vi "Section Page.vi"(8 "error in (no error)":errorcluster, 11 "Node Ptr":T1 format="%.0x") -> (0 "error out":errorcluster)   [LabVIEW 2019, in "Protection and Counter Addon System Explorer.lvlib"]
uses:
  Protection and Counter Addon System Explorer.lvlib
  <vilib>/NI VeriStand/Custom Device API/Custom Device Item Ref.ctl
  <vilib>/NI VeriStand/Custom Device API/Custom Device API.lvlib
panel:
  in  "SHDocVw.IWebBrowser2":refnum<k7>(container)
types:
  T1 = typedef "Custom Device API.lvlib/Custom Device Item Ref.ctl" = u64
  T2 = typedef "Custom Device API.lvlib/Custom Device Item Info.ctl" = cluster{"Name":string, "Is Channel":bool, "GUID":string, "Is Waveform":bool}
  T3 = typedef "Custom Device API.lvlib/Custom Device Commands.ctl" = enum16{"Default", "Item renamed", "Shutdown", "Dynamic button pressed"}
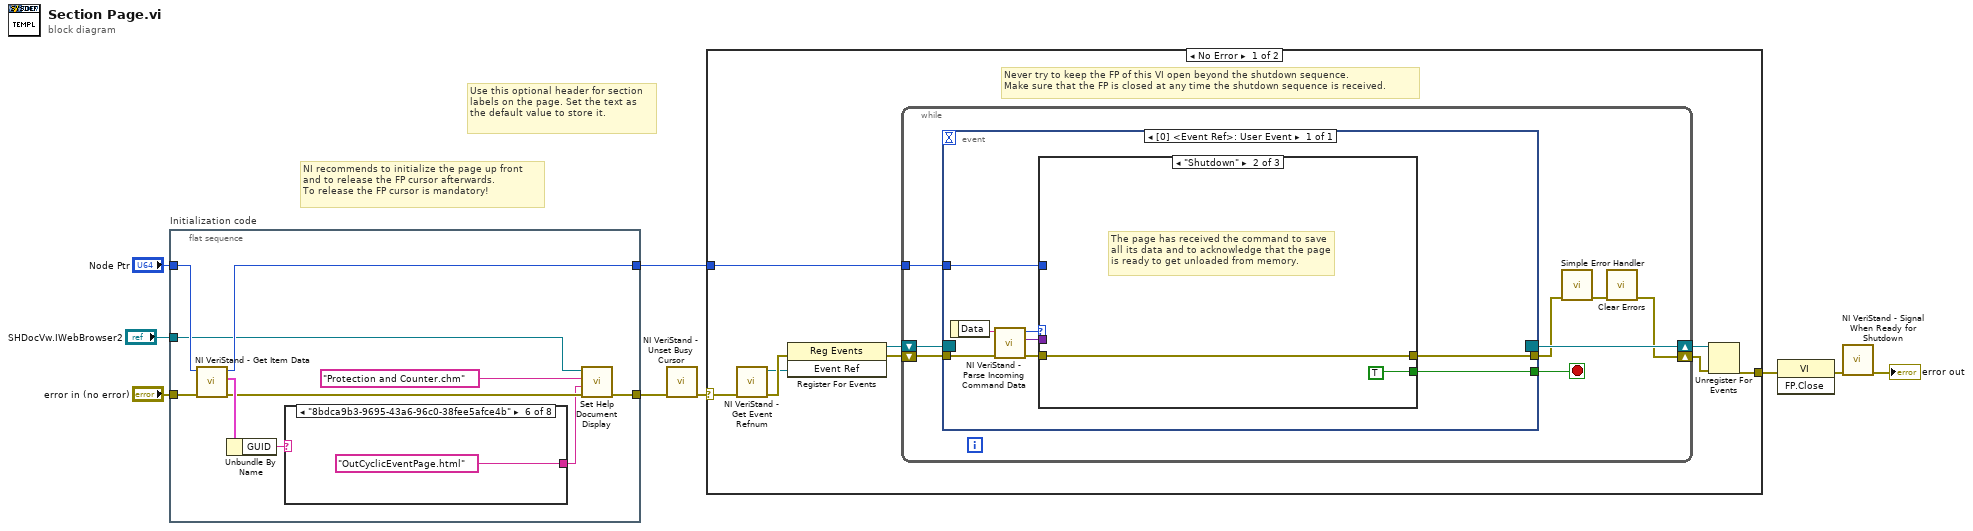
[diagram p0: block diagram]
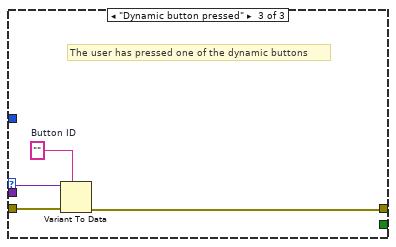
[diagram p3: hidden frame]
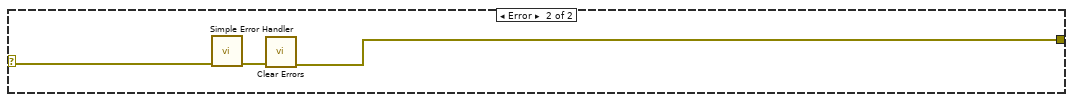
[diagram p4: hidden frame]
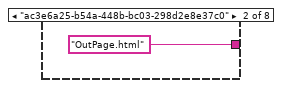
[diagram p6: hidden frame]
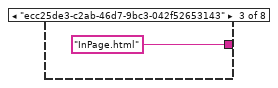
[diagram p7: hidden frame]
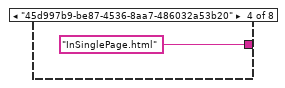
[diagram p8: hidden frame]
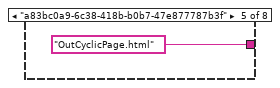
[diagram p9: hidden frame]
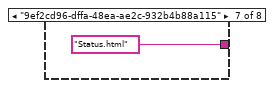
[diagram p10: hidden frame]
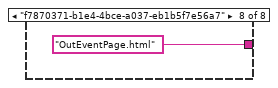
[diagram p11: hidden frame]
diagram:
  # "Use this optional header for section labels on the page. Set the text as the default value to store it."
  # "NI recommends to initialize the page up front\nand to release the FP cursor afterwards.\nTo release the FP cursor is mandatory!"
  n1 = flat-sequence "Initialization code" {
    tunnel: "error in (no error)" -> [w17]
    tunnel: "Node Ptr" -> [w19]
    tunnel: [w13] -> w5
    tunnel: [w18] -> w2
    tunnel: "SHDocVw.IWebBrowser2" -> [w10]
    frame #0 {
      n2 = call <vilib>:"NI VeriStand - Get Item Data.vi"("error in (no error)"=w17, "Item Ref in"=w19) -> ("error out"=w14:errorcluster, "Item Info"=w16:T2, "Item Ref out"=w18:T1)  [unwired: 6 in, 1 out]
      n3 = Unbundle By Name(w16) -> ("GUID"=w15:string)
      n4 = case shown="\"8bdca9b3-9695-43a6-96c0-38fee5afce4b\"" w15 {
        tunnel: [_ "OutPage.html" ("HTML File") "InPage.html" ("HTML File") "InSinglePage.html" ("HTML File") "OutCyclicPage.html" ("HTML File") "OutCyclicEventPage.html" ("HTML File") "Status.html" ("HTML File") "OutEventPage.html" ("HTML File")] -> w12
        frame Default {
        }
        frame "ac3e6a25-b54a-448b-bc03-298d2e8e37c0" {
        }
        frame "ecc25de3-c2ab-46d7-9bc3-042f52653143" {
        }
        frame "45d997b9-be87-4536-8aa7-486032a53b20" {
        }
        frame "a83bc0a9-6c38-418b-b0b7-47e877787b3f" {
        }
        frame "8bdca9b3-9695-43a6-96c0-38fee5afce4b" {
        }
        frame "9ef2cd96-dffa-48ea-ae2c-932b4b88a115" {
        }
        frame "f7870371-b1e4-4bce-a037-eb1b5f7e56a7" {
        }
      }
      n5 = call "Set Help Document Display.vi"("error in (no error)"=w14, "HTML File"=w12, "Main CHM File"="Protection and Counter.chm", "SHDocVw.IWebBrowser2"=w10) -> ("error out"=w13:errorcluster)  [unwired: 7 in]
    }
  }
  n6 = call <vilib>:"NI VeriStand - Unset Busy Cursor.vi"("error in (no error)"=w5) -> ("error out"=w4:errorcluster)  [unwired: 10 out]
  n7 = case shown="No Error" w4 {
    selector: w4 -> [w27 w61]
    tunnel: [w32 w59] -> w9
    tunnel: w2 -> [w28 _]
    frame No Error {
      # "Never try to keep the FP of this VI open beyond the shutdown sequence.\nMake sure that the FP is closed at any time the shutdown sequence is received."
      n8 = call <vilib>:"NI VeriStand - Get Event Refnum.vi"("error in (no error)"=w27) -> ("error out"=w35:errorcluster, "Event Ref"=w31:refnum<user-event>)  [unwired: 9 out]
      n9 = register-events(error in=w35, w31) -> (reference out=w29:refnum<event-registration>, error out=w30:errorcluster)  [unwired: 1 in]
      n10 = while {
        tunnel: w28 -> [w39]
        shift-right: [w36] -> w33
        shift-left: w30 -> [w42]
        shift-right: [w43] -> w34
        shift-left: w29 -> [w41]
        stop <- w40 stop-if-true
        n11 = event shown="[0] <Event Ref>: User Event" {
          selector: w41 -> [_]
          dyn-events: [_] -> w43
          timeout: _ -> [_]
          tunnel: w42 -> [w51]
          tunnel: [w47] -> w40
          tunnel: [w46] -> w38
          tunnel: w39 -> [w45]
          event User Event {
            n12 = event-data() -> ("Data"=w50:string)  [unwired: 1 out]
            n13 = call <vilib>:"NI VeriStand - Parse Incoming Command Data.vi"("error in (no error)"=w51, "Incoming data"=w50) -> ("error out"=w49:errorcluster, "Outgoing data"=w44:variant, "Action"=w48:T3)  [unwired: 7 out]
            n14 = case shown="\"Shutdown\"" w48 {
              tunnel: w49 -> [w52 w53 w58]
              tunnel: [_ TRUE _] -> w47
              tunnel: [w52 w53 w55] -> w46
              tunnel: w45 -> [_ _ _]
              tunnel: w44 -> [_ _ w57]
              frame "Default", Default {
              }
              frame "Shutdown" {
                # "The page has received the command to save all its data and to acknowledge that the page is ready to get unloaded from memory."
              }
              frame "Dynamic button pressed" {
                w56 = ""  # Button ID
                # "The user has pressed one of the dynamic buttons"
                n15 = Variant To Data(error in=w58, type=w56, Variant=w57) -> (error out=w55:errorcluster)  [unwired: 1 out]
              }
            }
          }
        }
        n16 = call <vilib>:"Simple Error Handler.vi"("error in (no error)"=w38) -> ("error out"=w37:errorcluster)  [unwired: 1 in, 7 out]
        n17 = call <vilib>:"Clear Errors.vi"("error in (no error)"=w37) -> ("error out"=w36:errorcluster)  [unwired: 1 in, 5 out]
      }
      n18 = Unregister For Events(event registration refnum=w34, error in=w33) -> (error out=w32:errorcluster)
    }
    frame Error {
      n19 = call <vilib>:"Simple Error Handler.vi"("error in (no error)"=w61) -> ("error out"=w60:errorcluster)  [unwired: 1 in, 7 out]
      n20 = call <vilib>:"Clear Errors.vi"("error in (no error)"=w60) -> ("error out"=w59:errorcluster)  [unwired: 1 in, 5 out]
    }
  }
  n21 = invoke class="VI" method="FP.Close"(error in=w9) -> (error out=w8:errorcluster)  [unwired: 2 in, 2 out]
  n22 = call <vilib>:"NI VeriStand - Signal When Ready for Shutdown.vi"("error in (no error)"=w8) -> ("error out"=→"error out":errorcluster)  [unwired: 10 out]
